vi "VectorField.vi"(4 "Properties":T1={"Color"=2147483647, "Arrow Scale"=nan, "Colormap"={"Map"=enum."Automatic", "Value Min"=nan, "Value Max"=nan, "Scaling"=enum."Default", "Reverse"=FALSE}, "Display"={"Alpha"=nan, "Z Order"=nan}} {"Color" items=["Automatic"=2147483647, "Black"=0, "White"=16777215, "Red"=16711680, "Green"=2263842, "Blue"=255, "Cyan"=65535, "Magenta"=16711935, "Yellow"=16776960]}, 5 "Y Vector Component":dbl[][](array[numeric]), 6 "Colormap Values":dbl[][](array[numeric]), 7 "X Vector Component":dbl[][](array[numeric]), 8 "error in (no error)":errorcluster, 9 "Y Coordinates":dbl[](array[numeric]), 10 "X Coordinates":dbl[](array[numeric]), 11 "Plot ID":T7 format="%x") -> (0 "error out":errorcluster, 3 "Plot ID Out":T7 format="%x")   [LabVIEW 2013, in "Advanced Plotting Toolkit.lvlib"]
doc: "Display a field of vector arrows."
uses:
  Advanced Plotting Toolkit.lvlib
  typedefs/PlotID.ctl
  VectorFieldProperties.ctl
  typedefs/PlotColor.ctl
  properties/Colormap.ctl
  properties/Colormap_Map.ctl
  properties/Colormap_Scaling.ctl
  properties/Display.ctl
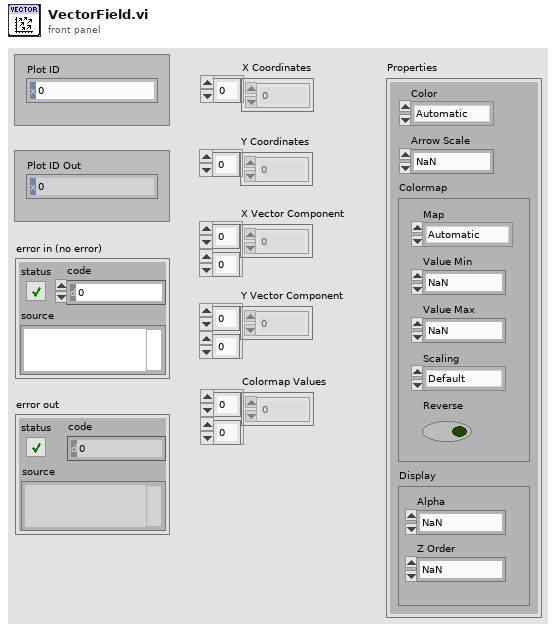
[diagram p1: front panel]
types:
  T1 = typedef "Advanced Plotting Toolkit.lvlib/VectorFieldProperties.ctl" = cluster{"Color":T2, "Arrow Scale":dbl, "Colormap":T3, "Display":T6}
  T2 = typedef "Advanced Plotting Toolkit.lvlib/PlotColor.ctl" = u32
  T3 = typedef "Advanced Plotting Toolkit.lvlib/Colormap.ctl" = cluster{"Map":T4, "Value Min":dbl, "Value Max":dbl, "Scaling":T5, "Reverse":bool}
  T4 = typedef "Advanced Plotting Toolkit.lvlib/Colormap_Map.ctl" = enum16{"Automatic", "Rainbow", "Hot and Cold", "White-Black", "White-Blue", "White-Green", "White-Red", "Fire", "Water", "Earth", "Air", "Pastel", "Banded", "Stepped"}
  T5 = typedef "Advanced Plotting Toolkit.lvlib/Colormap_Scaling.ctl" = enum16{"Default"}
  T6 = typedef "Advanced Plotting Toolkit.lvlib/Display.ctl" = cluster{"Alpha":dbl, "Z Order":dbl}
  T7 = typedef "Advanced Plotting Toolkit.lvlib/PlotID.ctl" = i32
  T8 = typedef "Advanced Plotting Toolkit.lvlib/KeyValue.ctl" = cluster{"Key":string, "Value":string}
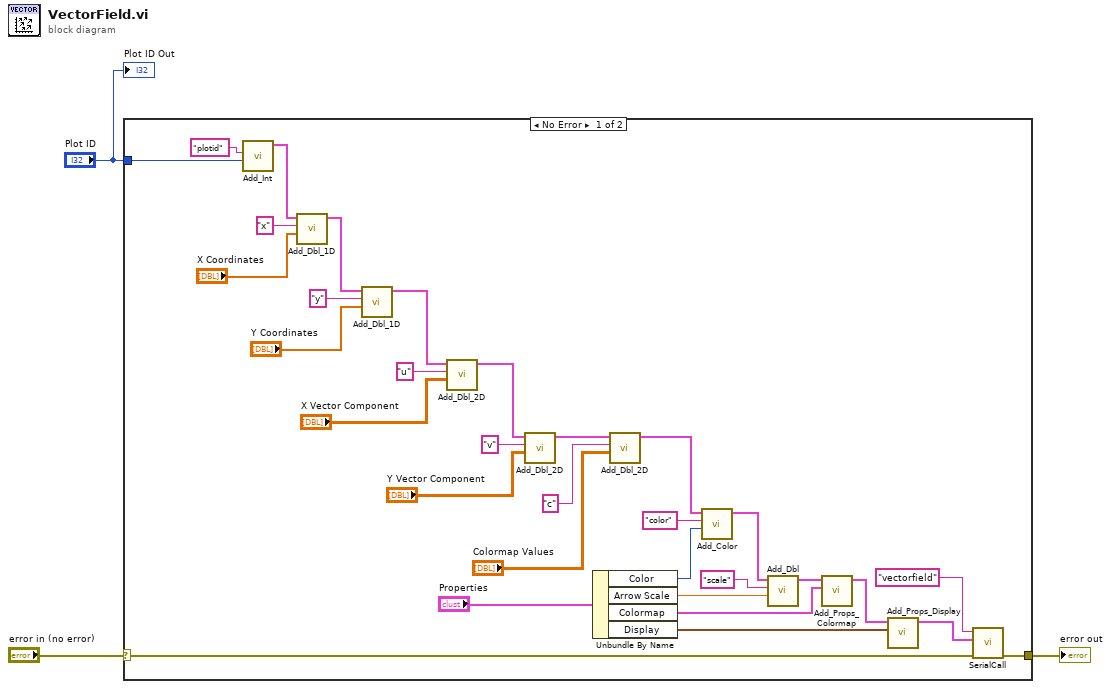
[diagram p0: block diagram]
diagram:
  n1 = case shown="No Error" "error in (no error)" {
    selector: "error in (no error)" -> [w11 w36]
    tunnel: "Plot ID" -> [w35 _]
    tunnel: [w10 w36] -> w1
    frame No Error {
      n2 = call "Add_Int.vi"("Value"=w35, "Key"="plotid") -> ("Keyword Array Out"=w33:T8[])  [unwired: 9 in]
      n3 = call "Add_Dbl_1D.vi"("Value"="X Coordinates", "Key"="x", "Keyword Array"=w33) -> ("Keyword Array Out"=w29:T8[])  [unwired: 8 in]
      n4 = call "Add_Dbl_1D.vi"("Value"="Y Coordinates", "Key"="y", "Keyword Array"=w29) -> ("Keyword Array Out"=w27:T8[])  [unwired: 8 in]
      n5 = call "Add_Dbl_2D.vi"("Value"="X Vector Component", "Key"="u", "Keyword Array"=w27) -> ("Keyword Array Out"=w23:T8[])  [unwired: 8 in]
      n6 = call "Add_Dbl_2D.vi"("Value"="Y Vector Component", "Key"="v", "Keyword Array"=w23) -> ("Keyword Array Out"=w21:T8[])  [unwired: 8 in]
      n7 = Unbundle By Name("Properties") -> ("Color"=w15:T2, "Arrow Scale"=w13:dbl, "Colormap"=w9:T3, "Display"=w6:T6)
      n8 = call "Add_Dbl_2D.vi"("Value"="Colormap Values", "Key"="c", "Keyword Array"=w21) -> ("Keyword Array Out"=w17:T8[])  [unwired: 8 in]
      n9 = call "Add_Color.vi"("Color"=w15, "Key"="color", "Keyword Array"=w17) -> ("Keyword Array Out"=w5:T8[])  [unwired: 8 in]
      n10 = call "Add_Dbl.vi"("Value"=w13, "Key"="scale", "Keyword Array"=w5) -> ("Keyword Array Out"=w4:T8[])  [unwired: 8 in]
      n11 = call "Add_Props_Colormap.vi"("Colormap"=w9, "Keyword Array"=w4) -> ("Keyword Array Out"=w8:T8[])  [unwired: 9 in]
      n12 = call "Add_Props_Display.vi"("Display"=w6, "Keyword Array"=w8) -> ("Keyword Array Out"=w7:T8[])  [unwired: 9 in]
      n13 = call "SerialCall.vi"("error in (no error)"=w11, "data"=w7, "Resource"="vectorfield") -> ("error out"=w10:errorcluster)  [unwired: 7 in, 1 out]
    }
    frame Error {
    }
  }
  "error out" <- w1
  "Plot ID Out" <- "Plot ID"
